vi "rotate phase angle of graph.vi"() -> ()   [LabVIEW 2009]
uses:
  <vilib>/imath/engines/lvmath2/RunTimeEngine/ErrorHandling/NIMS_Finalize Error.vi
  <vilib>/imath/engines/lvmath2/RunTimeEngine/Parser/MC_Version.vi
  <vilib>/imath/engines/lvmath2/RunTimeEngine/Managers/WorkSpace/UID Generator.vi
  <vilib>/imath/engines/lvmath2/RunTimeEngine/NodeEndStatement/NIMS_NodeEndStatement_Output.vi
  <instcachedir>/0/NIMS_NodeEndStatement_Output_53EC0D466D134D7ABD903AC30B43404B.lvgen/NIMS_NodeEndStatement_Output_53EC0D466D134D7ABD903AC30B43404B_000.vi
  <instcachedir>/0/NIMS_NodeEndStatement_Output_53EC0D466D134D7ABD903AC30B43404B.lvgen/NIMS_NodeEndStatement_Output_53EC0D466D134D7ABD903AC30B43404B_002.vi
  <vilib>/imath/engines/lvmath2/RunTimeEngine/Managers/SymbolTable/Clear UID.vi
  <vilib>/imath/engines/lvmath2/RunTimeEngine/LocalVariableDefStatement/MC_LocalVariableDefStatement_Display.vi
  <vilib>/imath/engines/lvmath2/RunTimeEngine/RunTimeType/NIMS_RunTimeType_From StrictType (excl LVString).vi
  <vilib>/Utility/file.llb/Write To Spreadsheet File (DBL).vi
  <vilib>/imath/engines/lvmath2/RunTimeEngine/Managers/SymbolTable/NIMS_WorkSpace.lvlib
  <vilib>/Analysis/NI_AALBase.lvlib
panel:
  out "3D array":dbl[][][](array[numeric])
  out "average of pages":dbl[][](array[numeric])
  out "#pages":i32
  out "#columns":i32
  out "#rows":i32
  in  "Put each data file you want to average into a separate array element":string[](array[string])
  in  "Read in from array":bool
  out "array of new data":dbl[][](array[numeric])
  in  "Output to file (pops up dialog box for name)":bool
  out "Theta 2":dbl
  in  "stop":bool
  out "Primary Graph 2":T1(graph) caption="cpsgraph"
  in  "Theta":dbl(knob) scale=0.0..360.0
  in  "Primary Graph":T2(graph)=[{"point array"=[{"x"=0.0, "y"=0.0}, {"x"=20.0, "y"=3.75511e-06}, {"x"=40.0, "y"=5.18563e-06}, {"x"=60.0, "y"=4.26176e-06}, {"x"=80.0, "y"=3.48689e-06}, {"x"=100.0, "y"=2.83124e-06}, {"x"=120.0, "y"=4.88761e-06}, {"x"=140.0, "y"=7.24199e-06}, {"x"=160.0, "y"=9.38779e-06}, {"x"=180.0, "y"=1.18614e-05}, {"x"=200.0, "y"=1.36197e-05}, {"x"=220.0, "y"=1.28747e-05}, {"x"=240.0, "y"=1.1921e-05}, {"x"=260.0, "y"=1.10865e-05}, {"x"=280.0, "y"=9.38779e-06}, {"x"=300.0, "y"=8.85135e-06}, {"x"=320.0, "y"=8.2851e-06}, {"x"=340.0, "y"=6.94397e-06}, {"x"=360.0, "y"=6.58634e-06}, {"x"=380.0, "y"=6.49694e-06}, {"x"=400.0, "y"=7.21219e-06}, {"x"=420.0, "y"=6.79496e-06}, {"x"=440.0, "y"=6.34792e-06}, {"x"=460.0, "y"=6.55654e-06}, {"x"=480.0, "y"=6.13931e-06}, {"x"=500.0, "y"=4.58959e-06}, {"x"=520.0, "y"=5.36445e-06}, {"x"=540.0, "y"=6.76516e-06}, {"x"=560.0, "y"=5.54326e-06}, {"x"=580.0, "y"=5.00682e-06}, {"x"=600.0, "y"=4.91741e-06}, {"x"=620.0, "y"=3.75511e-06}, {"x"=640.0, "y"=4.08295e-06}, {"x"=660.0, "y"=5.63267e-06}, {"x"=680.0, "y"=4.7982e-06}, {"x"=700.0, "y"=4.08295e-06}, {"x"=720.0, "y"=3.6657e-06}, {"x"=740.0, "y"=3.99354e-06}, {"x"=760.0, "y"=3.96374e-06}, {"x"=780.0, "y"=3.87433e-06}, {"x"=800.0, "y"=4.32137e-06}, {"x"=820.0, "y"=4.32137e-06}, {"x"=840.0, "y"=3.6061e-06}, {"x"=860.0, "y"=3.99354e-06}, {"x"=880.0, "y"=4.58959e-06}, {"x"=900.0, "y"=4.38097e-06}, {"x"=920.0, "y"=2.68222e-06}]}, {"point array"=[{"x"=0.0, "y"=0.0}, {"x"=20.0, "y"=1.54973e-06}, {"x"=40.0, "y"=1.37091e-06}, {"x"=60.0, "y"=1.34111e-06}, {"x"=80.0, "y"=3.87432e-07}, {"x"=100.0, "y"=7.15259e-07}, {"x"=120.0, "y"=9.53682e-07}, {"x"=140.0, "y"=2.47361e-06}, {"x"=160.0, "y"=2.98025e-06}, {"x"=180.0, "y"=4.35117e-06}, {"x"=200.0, "y"=3.7253e-06}, {"x"=220.0, "y"=3.96374e-06}, {"x"=240.0, "y"=2.92064e-06}, {"x"=260.0, "y"=1.75834e-06}, {"x"=280.0, "y"=1.81795e-06}, {"x"=300.0, "y"=2.86104e-06}, {"x"=320.0, "y"=2.56301e-06}, {"x"=340.0, "y"=2.14578e-06}, {"x"=360.0, "y"=2.20539e-06}, {"x"=380.0, "y"=1.78815e-06}, {"x"=400.0, "y"=7.74864e-07}, {"x"=420.0, "y"=6.55655e-07}, {"x"=440.0, "y"=5.9605e-07}, {"x"=460.0, "y"=6.55655e-07}, {"x"=480.0, "y"=1.1623e-06}, {"x"=500.0, "y"=6.55655e-07}, {"x"=520.0, "y"=1.90736e-06}, {"x"=540.0, "y"=1.31131e-06}, {"x"=560.0, "y"=1.2517e-06}, {"x"=580.0, "y"=8.94073e-07}, {"x"=600.0, "y"=1.57953e-06}, {"x"=620.0, "y"=1.10269e-06}, {"x"=640.0, "y"=8.94073e-07}, {"x"=660.0, "y"=1.1921e-07}, {"x"=680.0, "y"=-1.78815e-07}, {"x"=700.0, "y"=-9.23876e-07}, {"x"=720.0, "y"=-8.94074e-08}, {"x"=740.0, "y"=7.15259e-07}, {"x"=760.0, "y"=1.66894e-06}, {"x"=780.0, "y"=2.02657e-06}, {"x"=800.0, "y"=1.2219e-06}, {"x"=820.0, "y"=3.27827e-07}, {"x"=840.0, "y"=1.34111e-06}, {"x"=860.0, "y"=1.69874e-06}, {"x"=880.0, "y"=8.94073e-07}, {"x"=900.0, "y"=6.55655e-07}, {"x"=920.0, "y"=1.43052e-06}]}, {"point array"=[{"x"=0.0, "y"=0.0}, {"x"=20.0, "y"=4.08295e-06}, {"x"=40.0, "y"=5.36445e-06}, {"x"=60.0, "y"=4.47038e-06}, {"x"=80.0, "y"=3.51669e-06}, {"x"=100.0, "y"=2.92064e-06}, {"x"=120.0, "y"=4.97702e-06}, {"x"=140.0, "y"=7.65926e-06}, {"x"=160.0, "y"=9.86463e-06}, {"x"=180.0, "y"=1.26362e-05}, {"x"=200.0, "y"=1.41264e-05}, {"x"=220.0, "y"=1.34707e-05}, {"x"=240.0, "y"=1.22786e-05}, {"x"=260.0, "y"=1.12057e-05}, {"x"=280.0, "y"=9.59641e-06}, {"x"=300.0, "y"=9.29838e-06}, {"x"=320.0, "y"=8.67253e-06}, {"x"=340.0, "y"=7.2718e-06}, {"x"=360.0, "y"=6.94397e-06}, {"x"=380.0, "y"=6.76516e-06}, {"x"=400.0, "y"=7.24199e-06}, {"x"=420.0, "y"=6.82476e-06}, {"x"=440.0, "y"=6.37773e-06}, {"x"=460.0, "y"=6.61614e-06}, {"x"=480.0, "y"=6.25852e-06}, {"x"=500.0, "y"=4.64919e-06}, {"x"=520.0, "y"=5.69227e-06}, {"x"=540.0, "y"=6.91417e-06}, {"x"=560.0, "y"=5.69227e-06}, {"x"=580.0, "y"=5.09623e-06}, {"x"=600.0, "y"=5.15583e-06}, {"x"=620.0, "y"=3.90413e-06}, {"x"=640.0, "y"=4.17235e-06}, {"x"=660.0, "y"=5.63267e-06}, {"x"=680.0, "y"=4.7982e-06}, {"x"=700.0, "y"=4.17235e-06}, {"x"=720.0, "y"=3.6657e-06}, {"x"=740.0, "y"=4.05314e-06}, {"x"=760.0, "y"=4.29156e-06}, {"x"=780.0, "y"=4.38097e-06}, {"x"=800.0, "y"=4.50018e-06}, {"x"=820.0, "y"=4.32137e-06}, {"x"=840.0, "y"=3.84453e-06}, {"x"=860.0, "y"=4.32137e-06}, {"x"=880.0, "y"=4.67899e-06}, {"x"=900.0, "y"=4.44058e-06}, {"x"=920.0, "y"=3.03985e-06}]}] caption="cpsgraph"
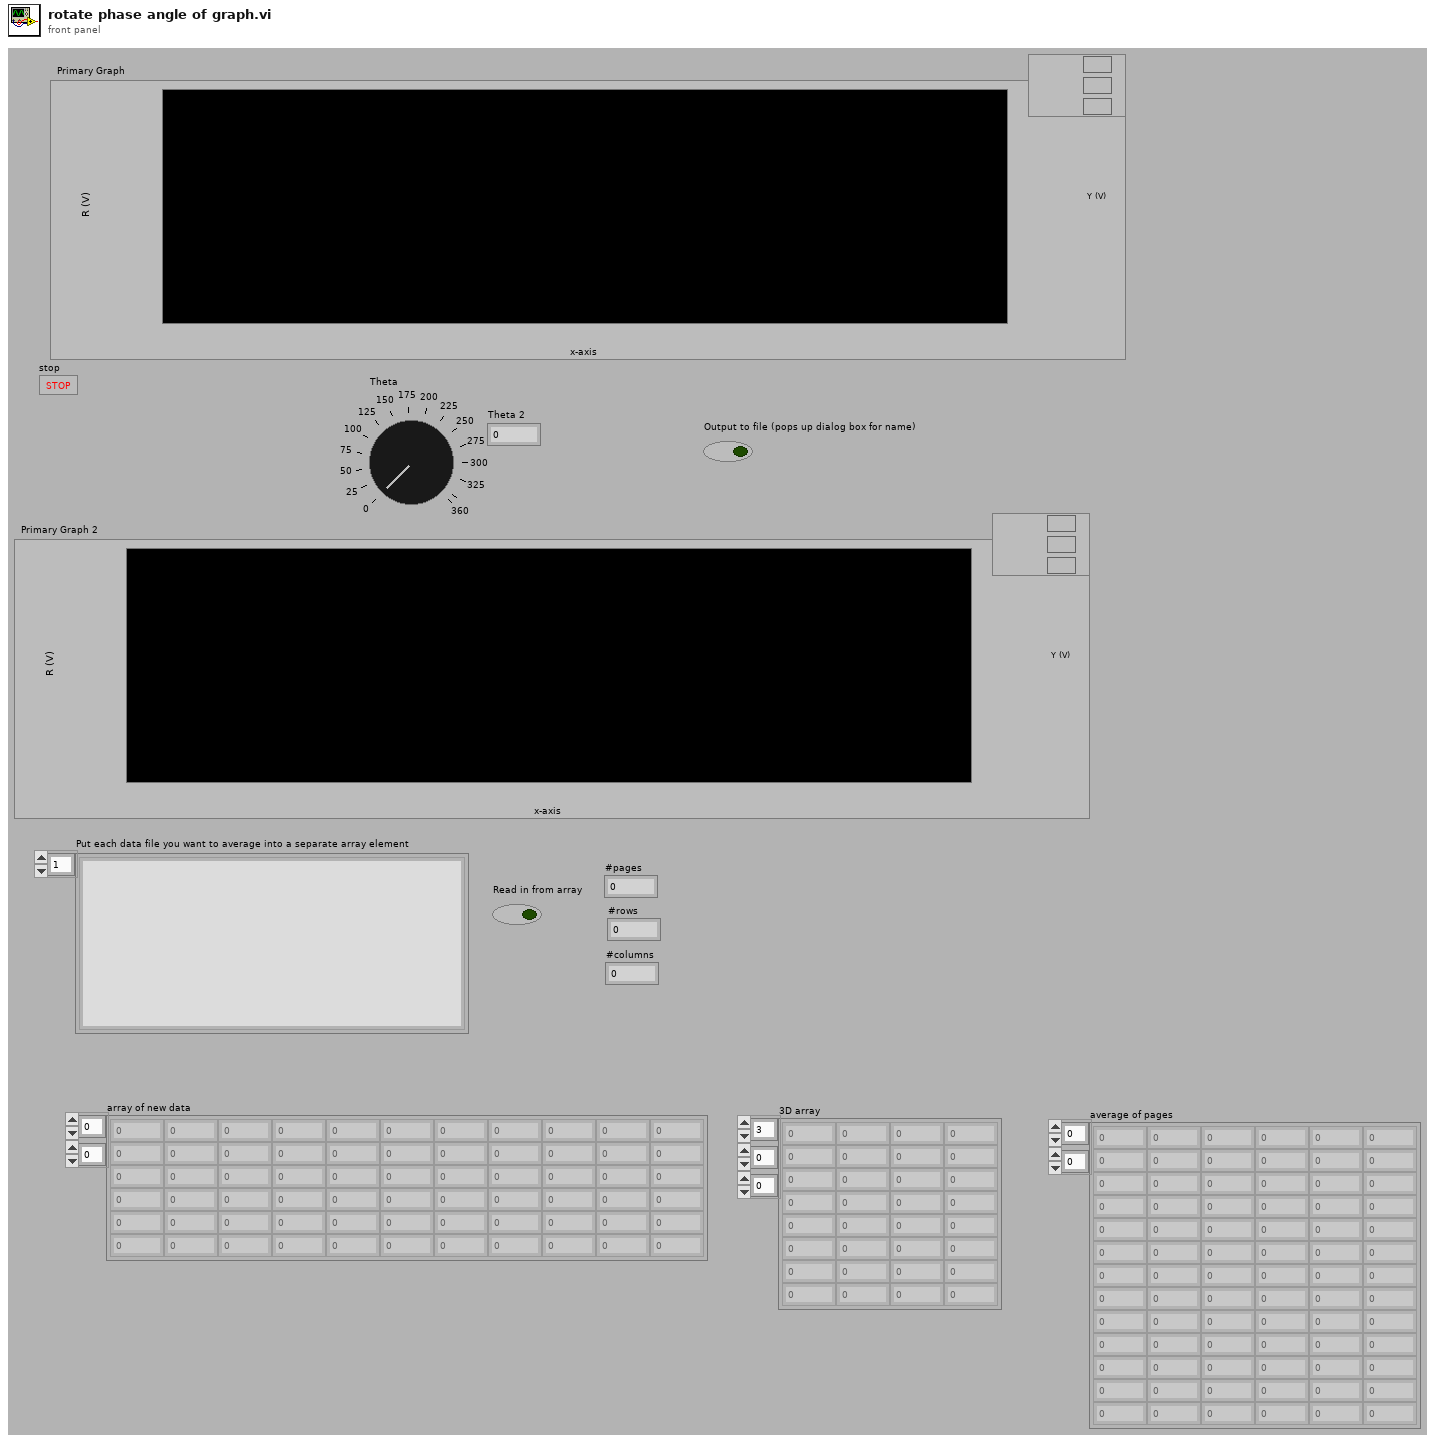
[diagram p1: front panel]
types:
  T1 = cluster{"point array":cluster{"x":dbl, "y":dbl}[]}[]
  T2 = typedef "Scan Driver.lvclass/Scan Graph.ctl" = cluster{"point array":cluster{"x":dbl, "y":dbl}[]}[]
  T3 = cluster{"Numeric 2":dbl, "Numeric 3":dbl, "Numeric 4":dbl}
  T4 = cluster{"point array":cluster{"x":dbl, "y":dbl}[]}
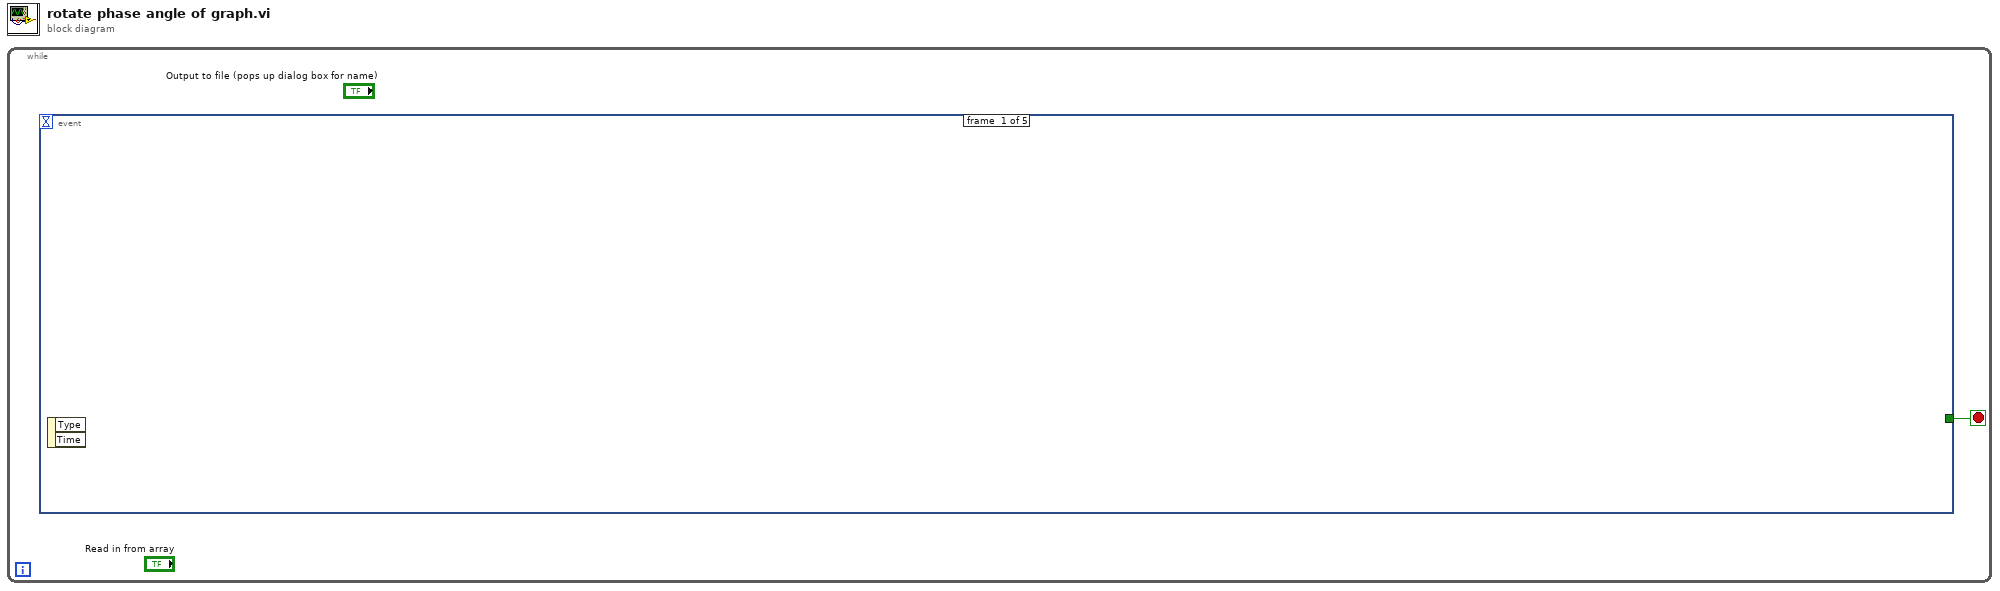
[diagram p0: block diagram]
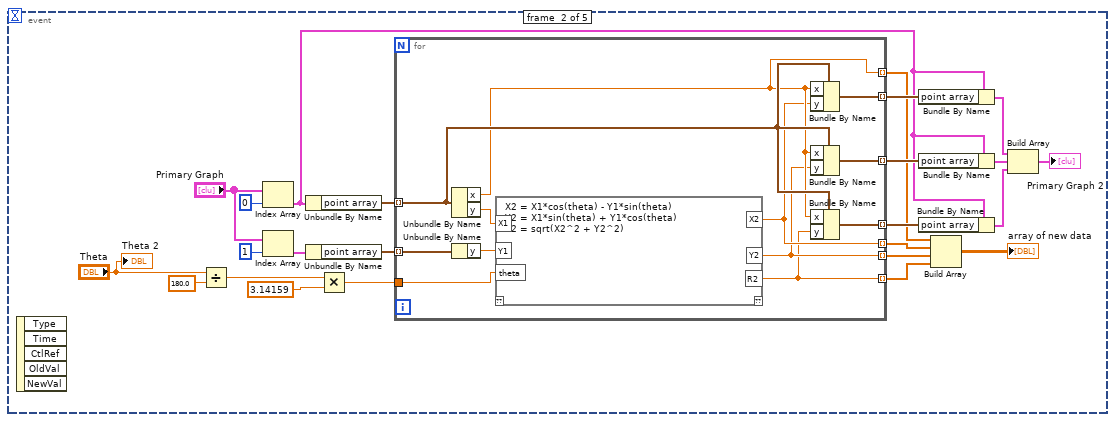
[diagram p2: hidden frame]
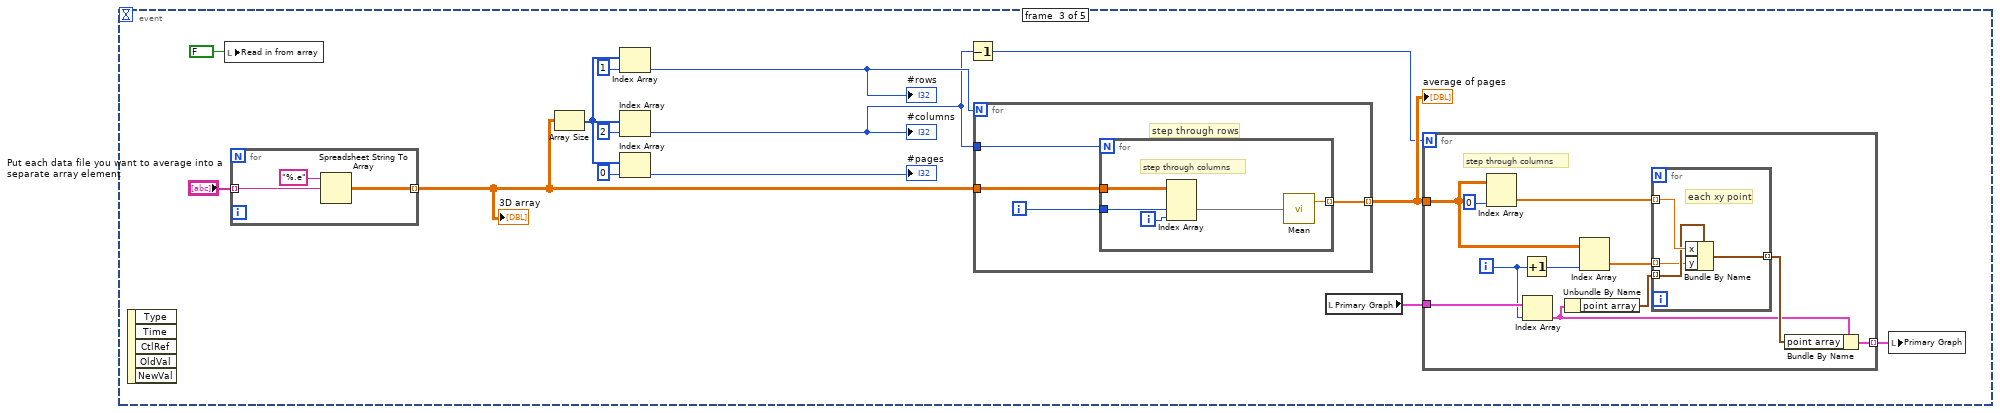
[diagram p3: hidden frame]
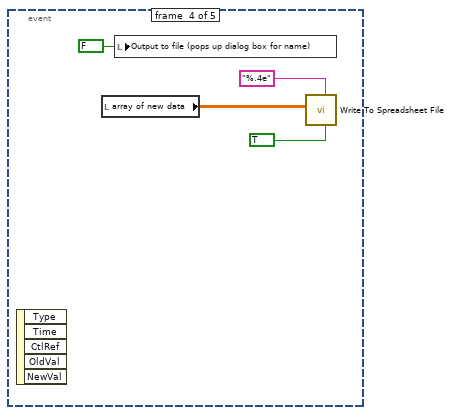
[diagram p4: hidden frame]
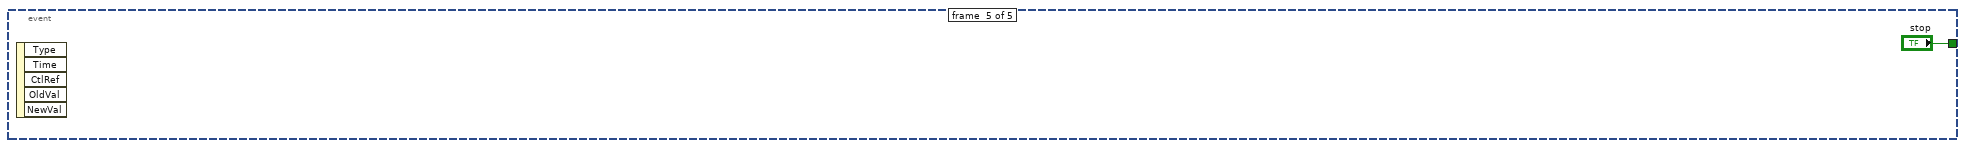
[diagram p5: hidden frame]
diagram:
  n1 = while {
    stop <- w1 stop-if-true
    n2 = event shown="[2] \"Read in from array\": Value Change" {
      selector: _ -> [_ _ _ _ _]
      dyn-events: _ -> [_ _ _ _ _]
      timeout: _ -> [_ _ _ _ _]
      tunnel: [_ _ _ _ "stop"] -> w1
      event #0 {
        n3 = event-data() -> ()  [unwired: 1 in, 2 out]
      }
      event #1 {
        n4 = event-data() -> ()  [unwired: 1 in, 5 out]
        n5 = Divide(x="Theta", y=180.0) -> (x/y=w15:dbl)
        n6 = Index Array(array="Primary Graph", index=0) -> (element=w18:T4)
        n7 = Index Array(array="Primary Graph", index=1) -> (element=w10:T4)
        n8 = Unbundle By Name(w18) -> ("point array"=w8:cluster{"x":dbl, "y":dbl}[])
        n9 = Unbundle By Name(w10) -> ("point array"=w11:cluster{"x":dbl, "y":dbl}[])
        n10 = Multiply(x=w15, y=3.14159) -> (x*y=w17:dbl)
        n11 = for {
          tunnel: w8 -> [w33] mode=indexing
          tunnel: w11 -> [w37] mode=indexing
          tunnel: w17 -> [w36]
          tunnel: [w32] -> w19 mode=indexing
          tunnel: [w31] -> w20 mode=indexing
          tunnel: [w30] -> w21 mode=indexing
          tunnel: [w29] -> w6 mode=indexing
          tunnel: [w28] -> w5 mode=indexing
          tunnel: [w27] -> w4 mode=indexing
          tunnel: [w26] -> w3 mode=indexing
          n12 = Unbundle By Name(w33) -> ("x"=w29:dbl, "y"=w35:dbl)
          n13 = Unbundle By Name(w37) -> ("y"=w34:dbl)
          n14 = mathscript code="X2 = X1*cos(theta) - Y1*sin(theta)\nY2 = X1*sin(theta) + Y1*cos(theta)\nR2 = sqrt(X2^2 + Y2^2)"("X1"=w35, "Y1"=w34, "theta"=w36) -> ("X2"=w28:dbl, "Y2"=w27:dbl, "R2"=w26:cdb)  [unwired: 2 out]
          n15 = Bundle By Name(cluster=w33, "x"=w29, "y"=w28) -> (w32:cluster{"x":dbl, "y":dbl})
          n16 = Bundle By Name(cluster=w33, "x"=w29, "y"=w27) -> (w31:cluster{"x":dbl, "y":dbl})
          n17 = Bundle By Name(cluster=w33, "x"=w29, "y"=w26) -> (w30:cluster{"x":dbl, "y":dbl})
        }
        n18 = Bundle By Name(cluster=w18, "point array"=w19) -> (w22:T4)
        n19 = Bundle By Name(cluster=w18, "point array"=w20) -> (w23:T4)
        n20 = Bundle By Name(cluster=w18, "point array"=w21) -> (w24:T4)
        n21 = Build Array(w6, w5, w4, w3) -> (→"array of new data":cdb[][])
        n22 = Build Array(w22, w23, w24) -> (→"Primary Graph 2":T1)
        "Theta 2" <- "Theta"
      }
      event #2 {
        n23 = event-data() -> ()  [unwired: 1 in, 5 out]
        n24 = local write "Read in from array"(FALSE ("Read in from array")) -> ()
        n25 = for {
          tunnel: "Put each data file you want to average into a separate array element" -> [w166] mode=indexing
          tunnel: [w165] -> w133 mode=indexing
          n26 = Spreadsheet String To Array(format string="%.e", spreadsheet string=w166) -> (array=w165:dbl[][])  [unwired: 2 in]
        }
        "3D array" <- w133
        n27 = Array Size(array=w133) -> (size(s)=w136:i32[])
        n28 = Index Array(array=w136, index=1) -> (element=w131:i32)
        "#rows" <- w131
        n29 = Index Array(array=w136, index=2) -> (element=w130:i32)
        "#columns" <- w130
        n30 = Index Array(array=w136, index=0) -> (element=→"#pages":i32)
        n31 = Decrement(x=w130) -> (x-1=w128:i32)
        n32 = for {
          N: w131 -> [_]
          tunnel: w133 -> [w158]
          tunnel: [w157] -> w129 mode=indexing
          tunnel: w130 -> [w156]
          i -> [w155]
          # "step through rows"
          n33 = for {
            N: w156 -> [_]
            tunnel: w158 -> [w162]
            tunnel: [w163] -> w157 mode=indexing
            tunnel: w155 -> [w161]
            i -> [w160]
            # "step through columns"
            n34 = Index Array(array=w162, index (dim 1)=w161, index (dim 2)=w160) -> (element=w159:dbl[])  [unwired: 1 in]
            n35 = call <vilib>:"Mean.vi"("X"=w159) -> ("mean"=w163:dbl)  [unwired: 1 out]
          }
        }
        "average of pages" <- w129
        n36 = local read "Primary Graph"() -> (w127:T2)
        n37 = for {
          N: w128 -> [_]
          tunnel: w129 -> [w150]
          tunnel: w127 -> [w142]
          tunnel: [w143] -> w126 mode=indexing
          i -> [w140]
          # "step through columns"
          n38 = Index Array(array=w150, index (col)=0 ("disabled index (col)")) -> (element=w147:dbl[])  [unwired: 1 in]
          n39 = Increment(x=w140) -> (x+1=w148:i32)
          n40 = Index Array(array=w142, index=w140) -> (element=w141:T4)
          n41 = Unbundle By Name(w141) -> ("point array"=w145:cluster{"x":dbl, "y":dbl}[])
          n42 = Index Array(array=w150, index (col)=w148) -> (element=w146:dbl[])  [unwired: 1 in]
          n43 = for {
            tunnel: w147 -> [w154] mode=indexing
            tunnel: w146 -> [w152] mode=indexing
            tunnel: w145 -> [w153] mode=indexing
            tunnel: [w151] -> w144 mode=indexing
            # "each xy point"
            n44 = Bundle By Name(cluster=w153, "x"=w154, "y"=w152) -> (w151:cluster{"x":dbl, "y":dbl})
          }
          n45 = Bundle By Name(cluster=w141, "point array"=w144) -> (w143:T4)
        }
        n46 = local write "Primary Graph"(w126) -> ()
      }
      event #3 {
        n47 = event-data() -> ()  [unwired: 1 in, 5 out]
        n48 = local read "array of new data"() -> (w169:dbl[][])
        n49 = local write "Output to file (pops up dialog box for name)"(FALSE ("Output to file")) -> ()
        n50 = call-poly <vilib>:"Write To Spreadsheet File.vi"("transpose? (no:F)"=TRUE, "format (%.3f)"="%.4e", "2D data"=w169) -> ()  [unwired: 5 in, 1 out]
      }
      event #4 {
        n51 = event-data() -> ()  [unwired: 1 in, 5 out]
      }
    }
  }
